vi "Dialog Trigger Settings.vi"(8 "error in (no error)":errorcluster, 11 "3300 in":refnum<class "3300.lvclass">) -> (0 "error out":errorcluster, 3 "3300 out":refnum<class "3300.lvclass">)   [LabVIEW 2019, in "3300.lvlib" / "3300.lvclass"]
uses:
  3300.lvclass
  builds/Instruments/Electronic Load.lvlibp/Custom Controls/Trigger Settings.ctl
  builds/Instruments/Electronic Load.lvlibp/Library/Electronic Load.lvclass
  builds/Instruments/Electronic Load.lvlibp/Custom Controls/E-Load Mode.ctl
panel:
  in  "Trigger Settings":T1={"Triggering"=FALSE, "Mode"=enum."Current", "Slew Rate"=0.0, "Transient"=0.0, "Initial"=0.0, "Samp Interval"=0.0, "Delay"=0.001, "Data Pts"=0, "Width"=0.0}
  in  "Cancel Button":bool
  in  "OK Button":bool
  in  "Triggered Channels":i32(listbox)
  in  "Move Down":bool
  in  "Move Up":bool
  in  "Remove":bool
  in  "Add":bool
  in  "Available Modules":u16(ring)
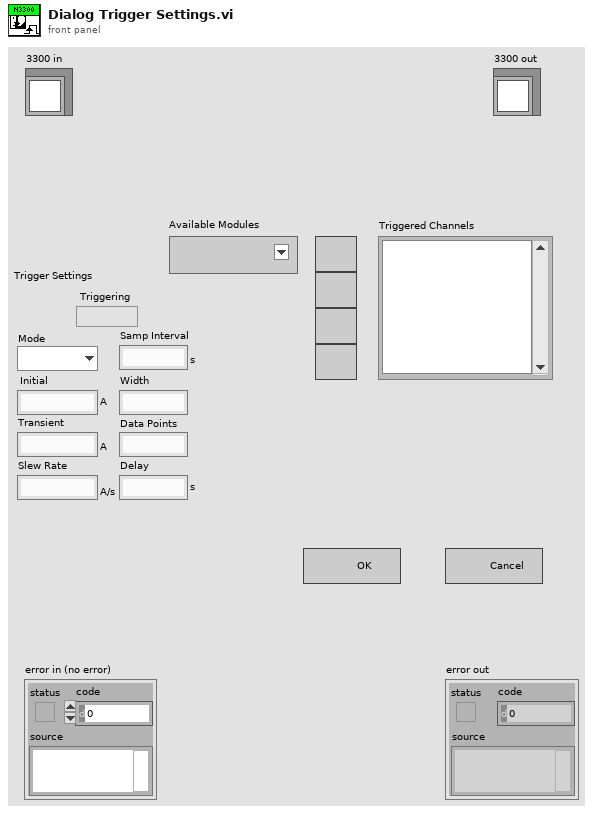
[diagram p1: front panel]
types:
  T1 = typedef "Electronic Load.lvlibp/Electronic Load.lvclass/Trigger Settings.ctl" = cluster{"Triggering":bool, "Mode":T2, "Slew Rate":dbl, "Transient":dbl, "Initial":dbl, "Samp Interval":dbl, "Delay":dbl, "Data Pts":i32, "Width":dbl}
  T2 = typedef "Electronic Load.lvlibp/Electronic Load.lvclass/E-Load Mode.ctl" = enum16{"Current", "Resistance", "Voltage"}
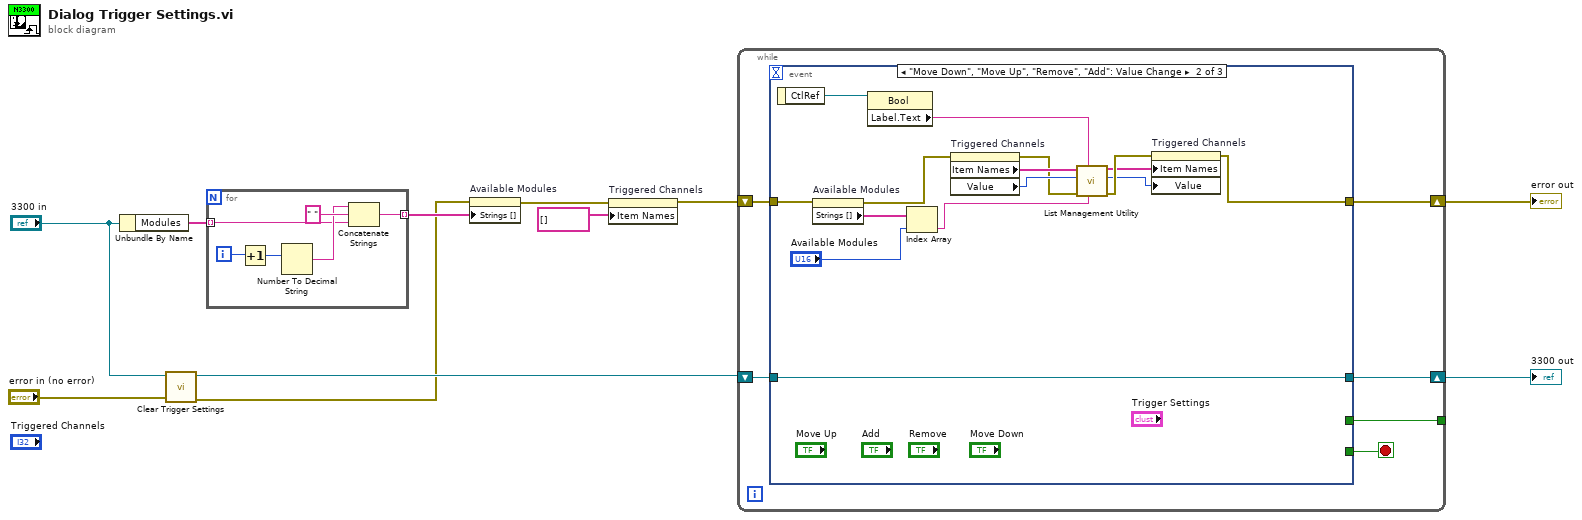
[diagram p0: block diagram]
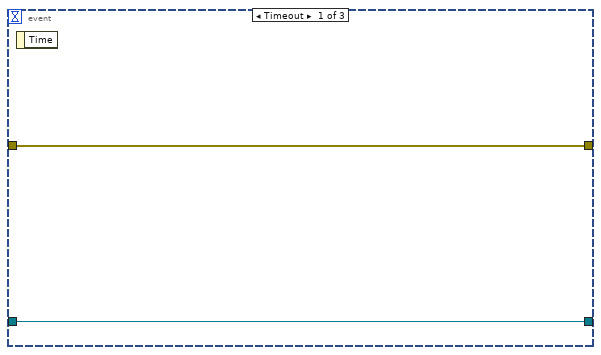
[diagram p2: hidden frame]
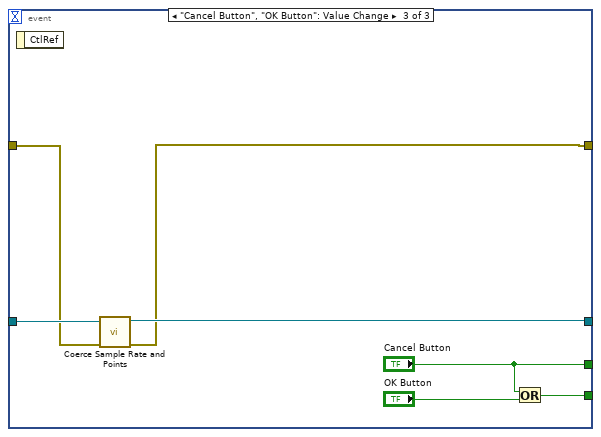
[diagram p3: hidden frame]
diagram:
  n1 = Unbundle By Name("3300 in") -> ("Modules"=w9:string[])
  n2 = call "Clear Trigger Settings.vi"("error in (no error)"="error in (no error)", "3300 in"="3300 in") -> ("error out"=w4:errorcluster, "3300 out"=w6:refnum<class "3300.lvclass">)  [unwired: 8 in]
  n3 = for {
    tunnel: w9 -> [w14] mode=indexing
    tunnel: [w13] -> w8 mode=indexing
    i -> [w12]
    n4 = Increment(x=w12) -> (x+1=w16:i32)
    n5 = Number To Decimal String(number=w16) -> (decimal integer string=w15:string)  [unwired: 1 in]
    n6 = Concatenate Strings(w15, " " ("string"), w14) -> (w13:string)
  }
  n7 = property on="Available Modules" class="Ring (strict)"(error in=w4, "Strings []"=w8) -> (error out=w2:errorcluster)  [unwired: 1 in, 1 out]
  n8 = property on="Triggered Channels" class="LstBox (strict)"(error in=w2, "Item Names"=string[] []) -> (error out=w3:errorcluster)  [unwired: 1 in, 1 out]
  n9 = while {
    shift-right: [w22] -> w11
    shift-left: w3 -> [w23]
    tunnel: [w20] -> _
    shift-right: [w18] -> w10
    shift-left: w6 -> [w19]
    stop <- w21 stop-if-true
    n10 = event shown="[1] \"Move Down\", \"Move Up\", \"Remove\", \"Add\": Value Change" {
      selector: _ -> [_ _ _]
      dyn-events: _ -> [_ _ _]
      timeout: _ -> [_ _ _]
      tunnel: w23 -> [w24 w39 w42]
      tunnel: [w24 w26 w41] -> w22
      tunnel: [_ _ w45] -> w21
      tunnel: [_ _ "Cancel Button"] -> w20
      tunnel: w19 -> [w25 w29 w44]
      tunnel: [w25 w29 w43] -> w18
      event Timeout {
        n11 = event-data() -> ()  [unwired: 1 in, 1 out]
      }
      event "Move Down", "Move Up", "Remove", "Add": Value Change {
        n12 = event-data() -> ("CtlRef"=w40:refnum<vi>)  [unwired: 1 in]
        n13 = property on="Available Modules" class="Ring (strict)"(error in=w39) -> (error out=w36:errorcluster, "Strings []"=w38:string[])  [unwired: 1 in, 1 out]
        n14 = property class="Bool"(reference=w40) -> ("Label.Text"=w27:string)  [unwired: 1 in, 2 out]
        n15 = Index Array(array=w38, index="Available Modules") -> (element=w37:string)
        n16 = property on="Triggered Channels" class="LstBox (strict)"(error in=w36) -> (error out=w33:errorcluster, "Item Names"=w35:string[], "Value"=w34:i32)  [unwired: 1 in, 1 out]
        n17 = call "List Management Utility.vi"("Item to add"=w37, "Action"=w27, "error in"=w33, "index"=w34, "Items In"=w35) -> ("error out 2"=w32:errorcluster, "Active Index"=w30:i32, "Items Out"=w31:string[])  [unwired: 4 in]
        n18 = property on="Triggered Channels" class="LstBox (strict)"(error in=w32, "Item Names"=w31, "Value"=w30) -> (error out=w26:errorcluster)  [unwired: 1 in, 1 out]
      }
      event "Cancel Button", "OK Button": Value Change {
        n19 = event-data() -> ()  [unwired: 1 in, 1 out]
        n20 = call "Coerce Sample Rate and Points.vi"("error in (no error)"=w42, "3300 in"=w44) -> ("error out"=w41:errorcluster, "3300 out"=w43:refnum<class "3300.lvclass">)  [unwired: 8 in]
        n21 = Or(x="Cancel Button", y="OK Button") -> (x .or. y?=w45:bool)
      }
    }
  }
  "error out" <- w11
  "3300 out" <- w10
